vi "Write LED INI File.vi"() -> ()   [LabVIEW 2018, in "LED Control Module.lvlib" / "LED INI File.lvlib"]
uses:
  LED INI File.lvlib
  INI File Control.ctl
  Public Controls/LVS Testplan.ctl
  Public Controls/LVS Instruments.ctl
  Public Controls/LVS Limits.ctl
  Public Controls/LVS Settings.ctl
  <vilib>/Utility/config.llb/NI_LVConfig.lvlib
  LED Control Module.lvlib
panel:
  out "error out":errorcluster
  in  "error in":errorcluster
  in  "LED INI Settings":T1={"TestPlan"={"Current Consumption"=TRUE, "Emission Spectrum"=TRUE}, "Instruments"={"Resistor 1"=1600.0, "Resistor 2"=390.0, "Resistor 3"=190.0}, "Limits"={"Current 1"=5.0, "Current 2"=20.0, "Current 3"=40.0, "Tolerance"=10.0, "Wavelength"=640.0}, "Settings"={"VLED 1"=2.0, "VLED 2"=2.2, "VLED 3"=2.4, "Source V"=10.0, "Result Path"=path "c:/temp"}} {"Settings"."Source V" format="%#_g V"; "Settings"."VLED 3" format="%#_g V"; "Settings"."VLED 2" format="%#_g V"; "Settings"."VLED 1" format="%#f V"; "Limits"."Wavelength" format="%#_g nm"; "Limits"."Tolerance" format="%#_g %"; "Limits"."Current 3" format="%#_g  mA"; "Limits"."Current 2" format="%#_g  mA"; "Limits"."Current 1" format="%#_g mA"; "Instruments"."Resistor 3" format="%#_g ohm"; "Instruments"."Resistor 2" format="%#_g ohm"; "Instruments"."Resistor 1" format="%#f ohm"}
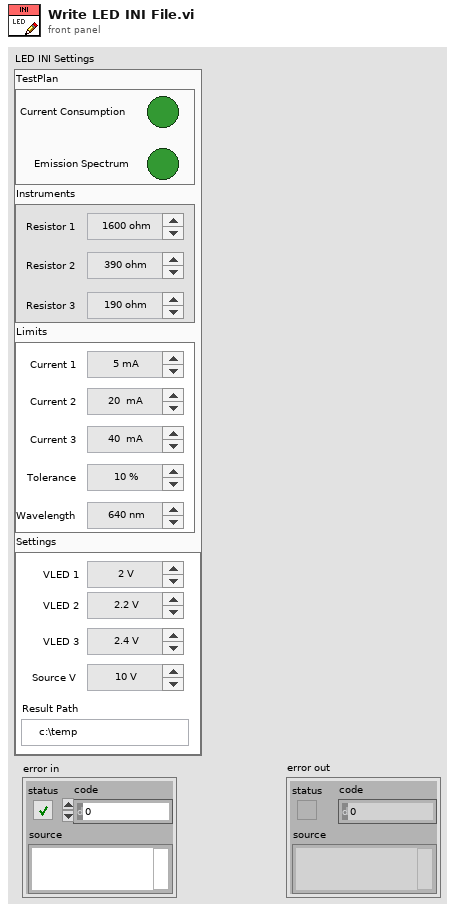
[diagram p1: front panel]
types:
  T1 = typedef "LED Control Module.lvlib/LED INI File.lvlib/INI File Control.ctl" = cluster{"TestPlan":T2, "Instruments":T3, "Limits":T4, "Settings":T5}
  T2 = typedef "LED Control Module.lvlib/LVS Testplan.ctl" = cluster{"Current Consumption":bool, "Emission Spectrum":bool}
  T3 = typedef "LED Control Module.lvlib/LVS Instruments.ctl" = cluster{"Resistor 1":dbl, "Resistor 2":dbl, "Resistor 3":dbl}
  T4 = typedef "LED Control Module.lvlib/LVS Limits.ctl" = cluster{"Current 1":dbl, "Current 2":dbl, "Current 3":dbl, "Tolerance":dbl, "Wavelength":dbl}
  T5 = typedef "LED Control Module.lvlib/LVS Settings.ctl" = cluster{"VLED 1":dbl, "VLED 2":dbl, "VLED 3":dbl, "Source V":dbl, "Result Path":path}
  T6 = enum32{"invalid app kind", "Development System", "Run Time System", "Student Edition", "Embedded LabVIEW", "Evaluation", "Custom"}
  T7 = typedef "NI_LVConfig.lvlib/Config Data RefNum.ctl" = refnum<k1>
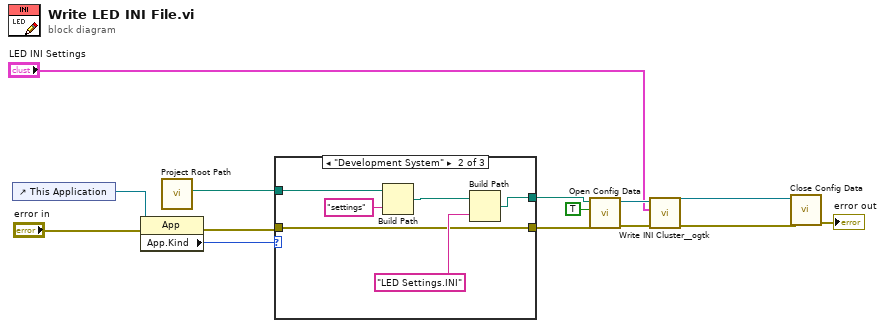
[diagram p0: block diagram]
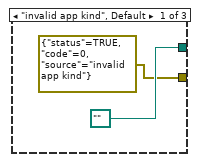
[diagram p2: hidden frame]
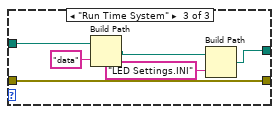
[diagram p3: hidden frame]
diagram:
  n1 = control-ref of="This Application"() -> (w14:refnum<vi>)
  n2 = property class="App"(reference=w14, error in="error in") -> (error out=w5:errorcluster, "App.Kind"=w13:T6)  [unwired: 1 out]
  n3 = call "Project Root Path.vi"() -> ("stripped path"=w12:path)  [unwired: 11 in]
  n4 = case shown="\"Development System\"" w13 {
    tunnel: w12 -> [_ w22 w28]
    tunnel: [path "" ("appended path") w18 w24] -> w8
    tunnel: [errorcluster {"status"=TRUE, "code"=0, "source"="invalid app kind"} ("error out") w17 w23] -> w6
    tunnel: w5 -> [_ w17 w23]
    frame "invalid app kind", Default {
    }
    frame "Development System" {
      n5 = Build Path(base path=w22, name or relative path="settings") -> (appended path=w20:path)
      n6 = Build Path(base path=w20, name or relative path="LED Settings.INI") -> (appended path=w18:path)
    }
    frame "Run Time System" {
      n7 = Build Path(base path=w28, name or relative path="data") -> (appended path=w25:path)
      n8 = Build Path(base path=w25, name or relative path="LED Settings.INI") -> (appended path=w24:path)
    }
  }
  n9 = call <vilib>:"Open Config Data.vi"("error in (no error)"=w6, "create file if necessary (T)"=TRUE, "configuration file path"=w8) -> ("error out"=w11:errorcluster, "refnum"=w10:T7)  [unwired: 6 in, 1 out]
  n10 = call <userlib>:"Write INI Cluster__ogtk.vi"("error in (no error)"=w11, "INI Fomatted Cluster"="LED INI Settings", "refnum"=w10) -> ("error out"=w3:errorcluster, "dup refnum"=w2:T7)  [unwired: 7 in]
  n11 = call <vilib>:"Close Config Data.vi"("error in (no error)"=w3, "refnum"=w2) -> ("error out"=→"error out":errorcluster)  [unwired: 8 in, 1 out]
